vi "Read Data.vi"(8 "error in (no error)":errorcluster, 11 "Model_AMC in":refnum<class "Model_AMC.lvclass">) -> (0 "error out":errorcluster, 3 "Model_AMC out":refnum<class "Model_AMC.lvclass">)   [LabVIEW 2021, in "Model_AMC.lvclass"]
uses:
  Model_AMC.lvclass
  Model_AMC.lvclass/Model_AMC.ctl
  <vilib>/ActorFramework/Actor/Actor.lvclass
  C:/Program Files (x86)/National Instruments/LabVIEW 2021/user.lib/John_Lib/AbstractActorTemplate/AbstractActorTemplate/UIActorTop.lvclass
  C:/Program Files (x86)/National Instruments/LabVIEW 2021/vi.lib/ActorFramework/Actor/Actor.lvclass
  C:/Program Files (x86)/National Instruments/LabVIEW 2021/project/Create Actor from Template/_Model_AMC/Model_AMC.lvclass
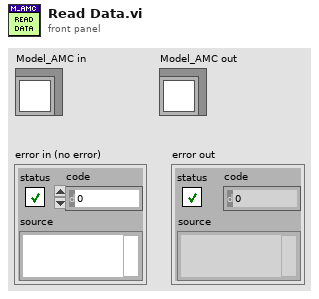
[diagram p1: front panel]
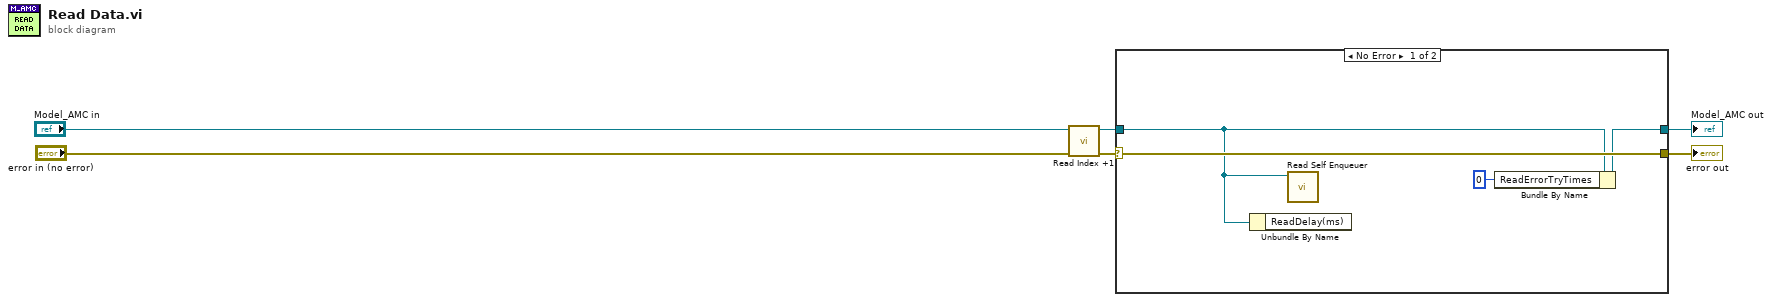
[diagram p0: block diagram]
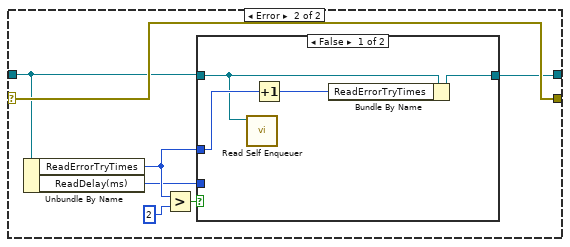
[diagram p2: hidden frame]
diagram:
  n1 = call "Read Index +1.vi"("error in (no error)"="error in (no error)", "Model_AMC in"="Model_AMC in") -> ("error out"=w2:errorcluster, "Model_AMC out"=w4:refnum<class "Model_AMC.lvclass">)  [unwired: 8 in]
  n2 = case shown="No Error" w2 {
    selector: w2 -> [w10 w17]
    tunnel: w4 -> [w7 w13]
    tunnel: [w9 w14] -> w3
    tunnel: [w10 w17] -> w1
    frame No Error {
      n3 = Unbundle By Name(w7) -> ()  [unwired: 1 out]
      n4 = call <vilib>:"Read Self Enqueuer.vi"("Actor"=w7) -> ()  [unwired: 10 in, 1 out]
      n5 = Bundle By Name(cluster=w7, "ReadErrorTryTimes"=u32 0) -> (w9:refnum<class "Model_AMC.lvclass">)
    }
    frame Error {
      n6 = Unbundle By Name(w13) -> ("ReadErrorTryTimes"=w12:u32, "ReadDelay(ms)"=w11:u32)
      n7 = Greater?(x=w12, y=u32 2) -> (0:w15:bool)
      n8 = case shown="False" w15 {
        tunnel: w11 -> [_ _]
        tunnel: [w21 w22] -> w14
        tunnel: w13 -> [w18 w22]
        tunnel: w12 -> [w20 _]
        frame False {
          n9 = call <vilib>:"Read Self Enqueuer.vi"("Actor"=w18) -> ()  [unwired: 10 in, 1 out]
          n10 = Increment(x=w20) -> (x+1=w19:u32)
          n11 = Bundle By Name(cluster=w18, "ReadErrorTryTimes"=w19) -> (w21:refnum<class "Model_AMC.lvclass">)
        }
        frame True {
        }
      }
    }
  }
  "error out" <- w1
  "Model_AMC out" <- w3
